vi "FL_Feedback_Node.vi"(1 "Reset Node":bool, 2 "Delay":u32, 4 "Input X":dbl format="%#_13g") -> (0 "Delayed X":dbl)   [LabVIEW 2018, in "Tracker.lvlib"]
doc: "This VI can accept both floating point and integer values."
uses:
  Tracker.lvlib
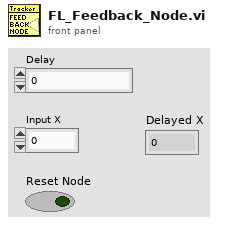
[diagram p1: front panel]
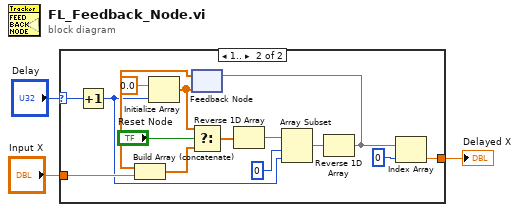
[diagram p0: block diagram]
diagram:
  n1 = case shown="1.." "Delay" {
    selector: "Delay" -> [_ w6]
    tunnel: "Input X" -> [w4 w17]
    tunnel: [w4 w10] -> w2
    frame 0, Default {
    }
    frame 1.. {
      n2 = Increment(x=w6) -> (x+1=w5:u32)
      n3 = Initialize Array(0.0, w5) -> (w7:dbl[])
      n4 = feedback #1(w7) -> (w18:dbl[])
      n5 = Build Array (concatenate)(w18, w17) -> (w16:dbl[])
      n6 = Select(t=w7, s="Reset Node", f=w16) -> (s? t:f=w9:dbl[])
      n7 = Reverse 1D Array(array=w9) -> (reversed array=w15:dbl[])
      n8 = Array Subset(array=w15, index=0, length=w5) -> (w13:dbl[])
      n9 = Reverse 1D Array(array=w13) -> (reversed array=w12:dbl[])
      n10 = feedback-in #1(w12) -> ()
      n11 = Index Array(array=w12, index=0) -> (element=w10:dbl)
    }
  }
  "Delayed X" <- w2
